vi "AM Initialize Hardware References.vi"(8 "error in (no error)":errorcluster, 10 "Message Data":variant, 11 "Hardware Resources in":T1) -> (0 "error out":errorcluster, 3 "Hardware Resources out":T1)   [LabVIEW 2020, in "OPC.lvlib"]
doc: "Initialize the hardware references."
uses:
  OPC.lvlib
  AM Configuration.ctl
  support/Message Queue/Message Cluster.ctl
  support/Message Queue/Message Queue.lvlib
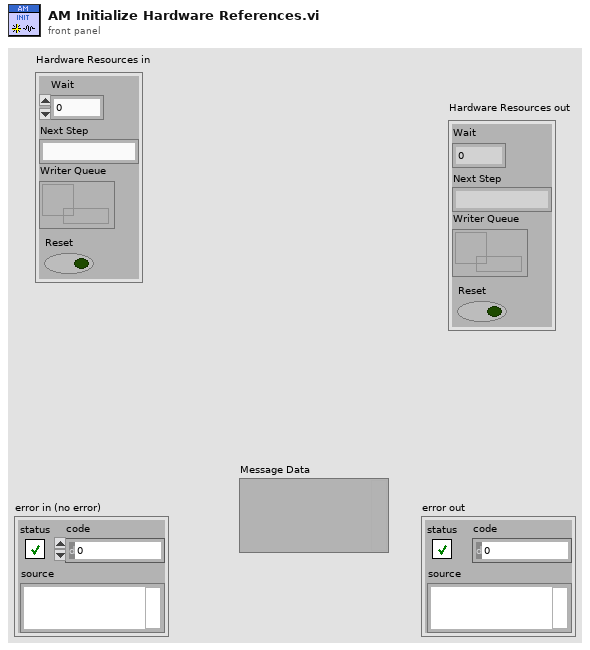
[diagram p1: front panel]
types:
  T1 = typedef "OPC.lvlib/AM Configuration.ctl" = cluster{"Wait":dbl, "Next Step":string, "Writer Queue":refnum<queue>, "Reset":bool}
  T2 = cluster{"Writer Queue":refnum<queue>, "Timeout":dbl}
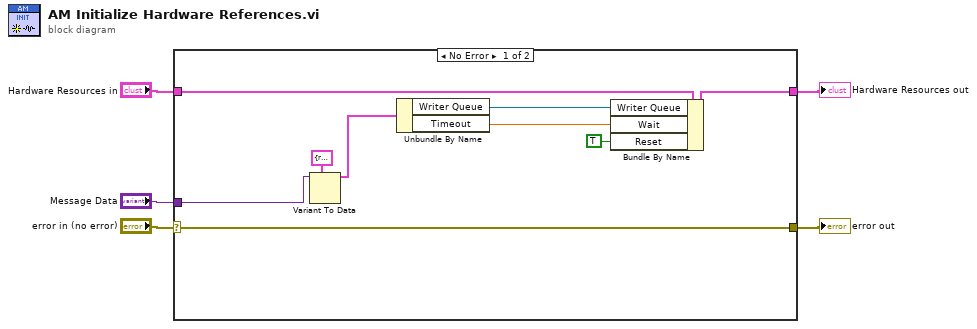
[diagram p0: block diagram]
diagram:
  n1 = case shown="No Error" "error in (no error)" {
    selector: "error in (no error)" -> [w13 w15]
    tunnel: [w13 w15] -> w4
    tunnel: "Hardware Resources in" -> [w14 w16]
    tunnel: [w11 w16] -> w1
    tunnel: "Message Data" -> [w12 _]
    frame No Error {
      n2 = Variant To Data(type=T2 {"Writer Queue"=refnum, "Timeout"=0.0}, Variant=w12) -> (data=w10:T2)  [unwired: 1 in, 1 out]
      n3 = Unbundle By Name(w10) -> ("Writer Queue"=w8:refnum<queue>, "Timeout"=w7:dbl)
      n4 = Bundle By Name(cluster=w14, "Writer Queue"=w8, "Wait"=w7, "Reset"=TRUE) -> (w11:T1)
    }
    frame Error {
    }
  }
  "Hardware Resources out" <- w1
  "error out" <- w4
